vi "shorefollow.vi"(2 "error in (no error)":errorcluster, 3 "Image in":T1) -> (0 "error out":errorcluster, 1 "Ordered Coordinates":i32[][](array[numeric]))   [LabVIEW 2014]
uses:
  <vilib>/vision/Image Controls.llb/IMAQ Image.ctl
panel:
  out "Path":T1(plugin-control)
  out "Original":T1(plugin-control)
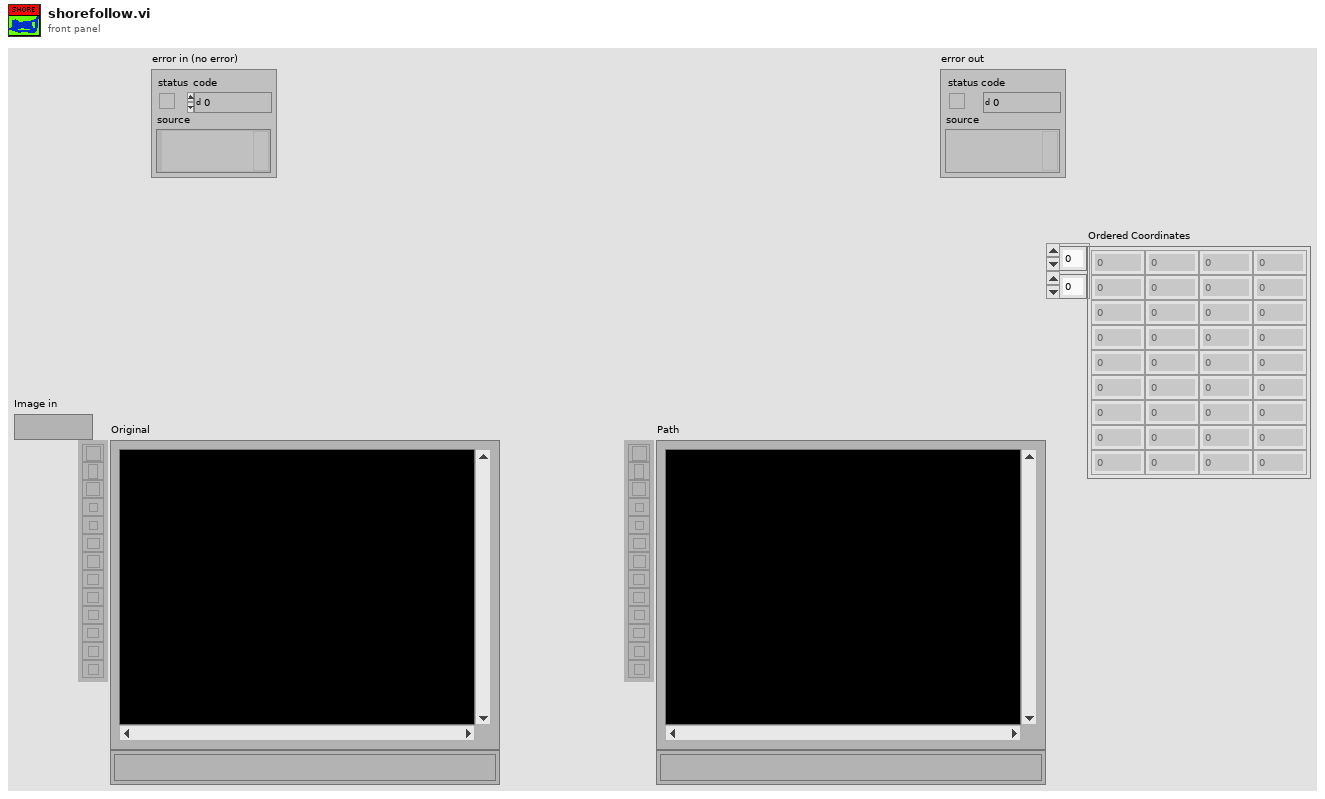
[diagram p1: front panel]
types:
  T1 = typedef "IMAQ Image.ctl" = refnum<image>
  T2 = typedef "Image Type" = u32
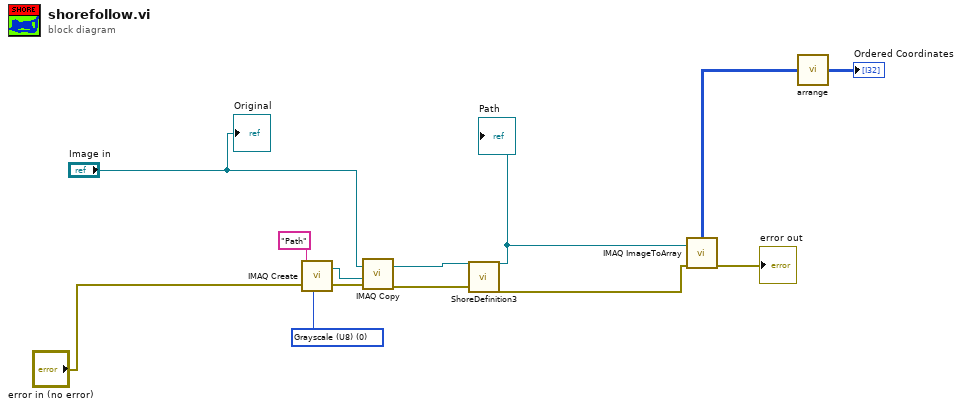
[diagram p0: block diagram]
diagram:
  w6 = T2 0 items=["Grayscale (U8)", "Grayscale (I16)", "Grayscale (SGL)", "Complex (CSG)", "RGB (U32)", "HSL (U32)", "RGB (U64)", "Grayscale (U16)"] ("Image Type")
  n1 = call "IMAQ Create"("Image Name"="Path", "Image Type"=w6, "error in (no error)"="error in (no error)") -> ("New Image"=w11:T1, "error out"=w12:errorcluster)  [unwired: 2 in]
  n2 = call "IMAQ Copy"("error in (no error)"=w12, "Image Dst"=w11, "Image Src"="Image in") -> ("error out"=w9:errorcluster, "Image Dst Out"=w10:T1)  [unwired: 3 in]
  n3 = call "ShoreDefinition3.vi"("Image In"=w10, "error in"=w9) -> ("Image Out"=w8:T1, "error out"=w7:errorcluster)  [unwired: 24 in]
  "Path" <- w8
  n4 = call "IMAQ ImageToArray"("error in (no error)"=w7, "Image"=w8) -> ("error out"=→"error out":errorcluster, "Image Pixels (U8)"=w5:u8[][])  [unwired: 2 in, 3 out]
  n5 = call "arrange.vi"("Input Array"=w5) -> ("Ordered Coordinates"=→"Ordered Coordinates":i32[][])
  "Original" <- "Image in"
